vi "Read beeing pushed.vi"(8 "error in (no error)":errorcluster, 11 "GameObject in":refnum<class "GameObject.lvclass">) -> (0 "error out":errorcluster, 2 "beeing pushed":bool, 3 "GameObject out":refnum<class "GameObject.lvclass">)   [LabVIEW 2019, in "RT_Game.lvlib" / "GameObject.lvclass"]
uses:
  GameObject.lvclass
  GameObject.lvclass/GameObject.ctl
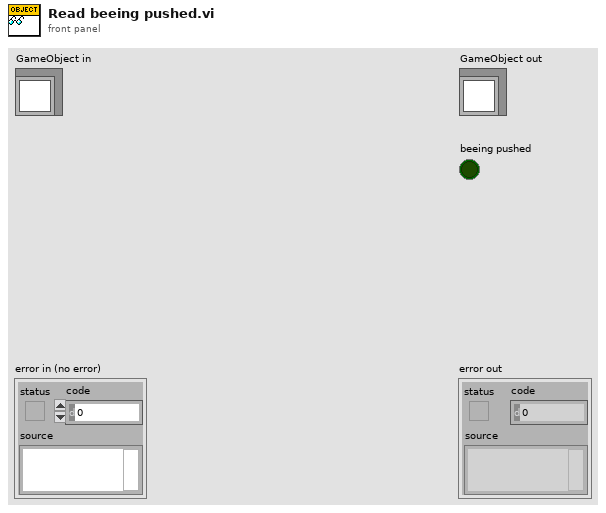
[diagram p1: front panel]
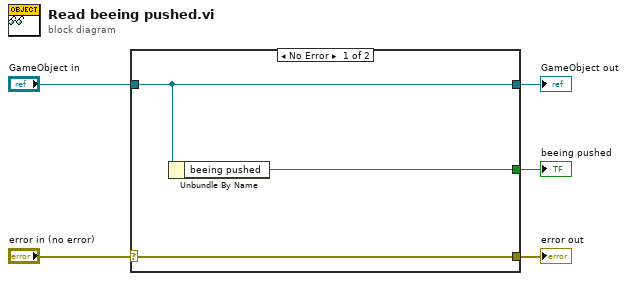
[diagram p0: block diagram]
diagram:
  n1 = case shown="No Error" "error in (no error)" {
    selector: "error in (no error)" -> [w8 w9]
    tunnel: [w8 w9] -> w4
    tunnel: [w7 w10] -> w2
    tunnel: "GameObject in" -> [w7 w10]
    tunnel: [w6 _] -> w1
    frame No Error {
      n2 = Unbundle By Name(w7) -> ("beeing pushed"=w6:bool)
    }
    frame Error {
    }
  }
  "error out" <- w4
  "GameObject out" <- w2
  "beeing pushed" <- w1
